vi "Stop.vi"(6 "timeout in ms (-1)":i32=-1, 8 "error in (no error)":errorcluster, 10 "Shared Key":string, 11 "SMO":refnum<class "SMO.lvclass">) -> (0 "error out":errorcluster, 3 "SMO out":refnum<class "SMO.lvclass">)   [LabVIEW 2021, in "smo.lvlib" / "SMO.lvclass"]
doc: "This method signal all the running processes to shutdown.\n\n<b>ms timeout</b> is the max amount of time allowed for the process to shutdown before an error is reported. <b>ms timeout</b> default is -1 = never times out\n\nNote 01: This method is overridable by descendant\nNote 02: When overridden, Call Parent Method is required\n\n---------------------------------------------------------------\nJKI State Machine Objects™\nhttp://jki.net/state-machine-objects/\nCopyright (C) 2005-2015, JKI <info@jki.net>\nALL RIGHTS RESERVED"
uses:
  SMO.lvclass
  SMO.lvclass/SMO.ctl
  Support/Attribute.Owner/Attribute.Owner.lvclass/Attribute.Owner.ctl
  Support/Attribute.Owner/Verify Key Match.vi
  Private/GetVariant(Attr).vi
  Support/Attribute.Owner/Read Shared Key.vi
  Private/ReftoDVR--SMO.vi
  Support/Attribute.Owner/Attribute.Owner.lvclass
panel:
  # "For instructions on how to use the JKI State Machine Objects, examples and video tutorials, visit:\nhttp://jki.net/state-machine-objects/\n\nJKI State Machine Objects™\nhttp://jki.net/state-machine-objects/\nCopyright (C) 2005-2015, JKI <info@jki.net>\nALL RIGHTS RESERVED"
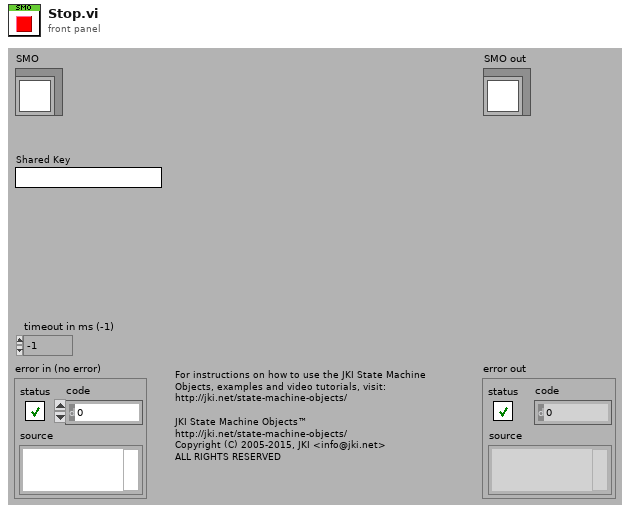
[diagram p1: front panel]
types:
  T1 = typedef "smo.lvlib/SMO.lvclass/SMOState --Enum.ctl" = enum16{"unknown", "Created", "Started", "Stopped"}
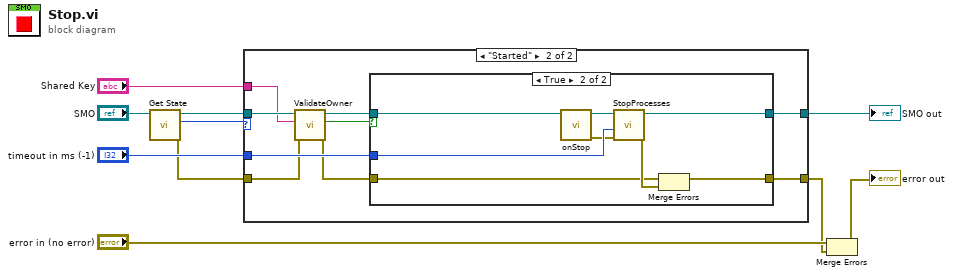
[diagram p0: block diagram]
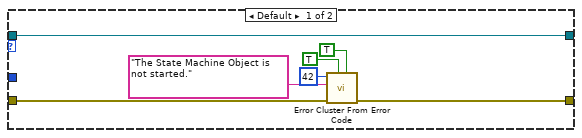
[diagram p2: hidden frame]
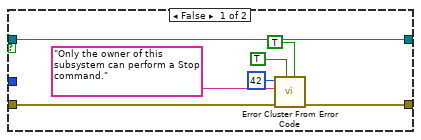
[diagram p3: hidden frame]
diagram:
  n1 = call "Get State.vi"("SMO"="SMO") -> ("error out"=w4:errorcluster, "SMO State"=w6:T1, "SMO out"=w7:refnum<class "SMO.lvclass">)  [unwired: 8 in]
  n2 = case shown="\"Started\"" w6 {
    tunnel: [w17 w26] -> w10
    tunnel: "timeout in ms (-1)" -> [_ w25]
    tunnel: [w11 w24] -> w1
    tunnel: w7 -> [w17 w23]
    tunnel: w4 -> [w13 w19]
    tunnel: "Shared Key" -> [_ w20]
    frame Default {
      n3 = call <vilib>:"Error Cluster From Error Code.vi"("is warning? (False)"=TRUE, "show call chain? (False)"=TRUE, "error in (no error)"=w13, "error message (\"\")"="The State Machine Object is not started." ("source"), "error code (0)"=42) -> ("error out"=w11:errorcluster)  [unwired: 4 in]
    }
    frame "Started" {
      n4 = call "ValidateOwner.vi"("error in (no error)"=w19, "Shared Key"=w20, "SMO in"=w23) -> ("error out"=w18:errorcluster, "key matched"=w21:bool, "SMO out"=w22:refnum<class "SMO.lvclass">)  [unwired: 5 in, 1 out]
      n5 = case shown="True" w21 {
        tunnel: [w33 w41] -> w26
        tunnel: w25 -> [_ w40]
        tunnel: [w28 w39] -> w24
        tunnel: w18 -> [w27 w35]
        tunnel: w22 -> [w33 w34]
        frame False {
          n6 = call <vilib>:"Error Cluster From Error Code.vi"("is warning? (False)"=TRUE, "show call chain? (False)"=TRUE, "error in (no error)"=w27, "error message (\"\")"="Only the owner of this subsystem can perform a Stop command." ("source"), "error code (0)"=42) -> ("error out"=w28:errorcluster)  [unwired: 4 in]
        }
        frame True {
          n7 = call-dynamic "onStop.vi"("SMO"=w34) -> ("error out"=w36:errorcluster, "SMO out"=w38:refnum<class "SMO.lvclass">)  [unwired: 9 in]
          n8 = call "StopProcesses.vi"("error in (no error)"=w36, "timeout in ms (-1)"=w40, "SMO"=w38) -> ("error out"=w37:errorcluster, "SMO out"=w41:refnum<class "SMO.lvclass">)  [unwired: 7 in]
          n9 = Merge Errors(w35, w37) -> (w39:errorcluster)
        }
      }
    }
  }
  "SMO out" <- w10
  n10 = Merge Errors("error in (no error)", w1) -> (→"error out":errorcluster)
